vi "Angle between Pts.vi"(10 "Pt 2":cluster{"x":dbl, "y":dbl, "th":dbl}, 11 "Pt 1":cluster{dbl, dbl, i32}) -> (2 "Distance ft":dbl, 3 "Angle rad":dbl)   [LabVIEW 2025]
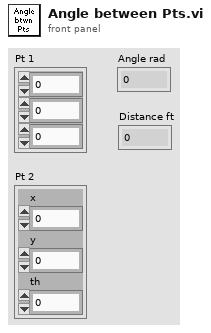
[diagram p1: front panel]
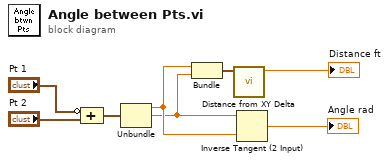
[diagram p0: block diagram]
diagram:
  n1 = Compound Arithmetic op=ADD(invert "Pt 1", "Pt 2") -> (w5:cluster{dbl, dbl, dbl})
  n2 = Unbundle(w5) -> (w4:dbl, w3:dbl)  [unwired: 1 out]
  n3 = Bundle(w4, w3) -> (w2:cluster{dbl, dbl})  [unwired: 1 in]
  n4 = call "Distance from XY Delta.vi"("Delta Point"=w2) -> ("Distance"=→"Distance ft":dbl)  [unwired: 10 in]
  n5 = Inverse Tangent (2 Input)(1:w4, 2:w3) -> (0:→"Angle rad":dbl)
